vi "Handle Sink Event.vi"(8 "error in (no error)":errorcluster, 10 "Event Data":refnum<class "Event.lvclass">, 11 "Event Source in":refnum<class "Event Source.lvclass">) -> (0 "error out":errorcluster, 3 "Event Source out":refnum<class "Event Source.lvclass">)   [LabVIEW 2016, in "Event Source.lvlib" / "Event Source.lvclass"]
uses:
  Event Source.lvclass
  Event/Event.lvclass
  Event Source Messages/Receive and Broadcast Event Msg/Receive and Broadcast Event Msg.lvclass
  Event Source.lvclass/Event Source.ctl
  Event Source Messages/Abstract Source Event Handler/Abstract Source Event Handler.lvclass
panel:
  in  "Receive and Broadcast Event Msg in":refnum<class "Receive and Broadcast Event Msg.lvclass">
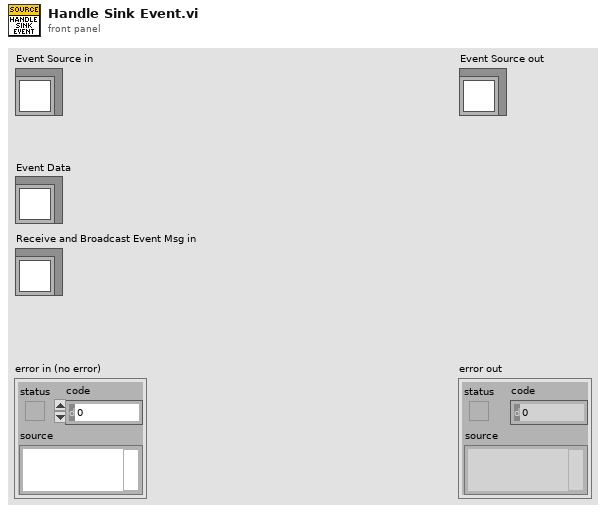
[diagram p1: front panel]
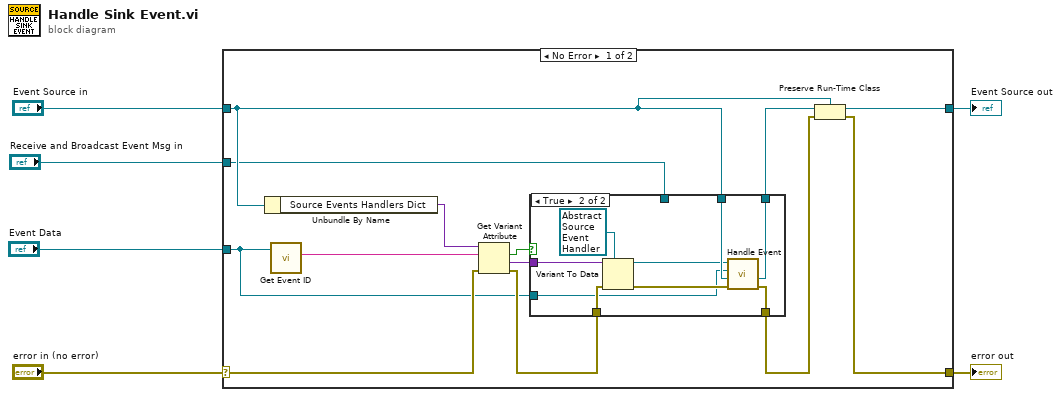
[diagram p0: block diagram]
diagram:
  n1 = case shown="No Error" "error in (no error)" {
    selector: "error in (no error)" -> [w15 w32]
    tunnel: [w9 w32] -> w5
    tunnel: [w12 w31] -> w2
    tunnel: "Event Source in" -> [w11 w31]
    tunnel: "Event Data" -> [w7 _]
    tunnel: "Receive and Broadcast Event Msg in" -> [w8 _]
    frame No Error {
      n2 = Unbundle By Name(w11) -> ("Source Events Handlers Dict"=w19:variant)
      n3 = call-dynamic "Get Event ID.vi"("Event in"=w7) -> ("Event ID"=w18:string)  [unwired: 8 in, 2 out]
      n4 = Get Variant Attribute(Variant=w19, name=w18, error in=w15) -> (found=w17:bool, value=w16:variant, error out=w14:errorcluster)  [unwired: 1 in, 1 out]
      n5 = case shown="True" w17 {
        tunnel: w16 -> [_ w30]
        tunnel: w14 -> [w21 w28]
        tunnel: w11 -> [w20 w24]
        tunnel: [w20 w27] -> w13
        tunnel: [w21 w26] -> w10
        tunnel: w8 -> [_ _]
        tunnel: w7 -> [_ w23]
        frame False {
        }
        frame True {
          n6 = Variant To Data(error in=w28, type=refnum<class "Abstract Source Event Handler.lvclass"> refnum ("Source Event Fire Handler"), Variant=w30) -> (data=w22:refnum<class "Abstract Source Event Handler.lvclass">, error out=w25:errorcluster)
          n7 = call-dynamic "Handle Event.vi"("error in (no error)"=w25, "Event Source in"=w24, "Event Data"=w23, "Abstract Source Event Handler in"=w22) -> ("error out"=w26:errorcluster, "Event Source out"=w27:refnum<class "Event Source.lvclass">)  [unwired: 5 in, 1 out]
        }
      }
      n8 = Preserve Run-Time Class(object in=w13, error in=w10, 2:w11) -> (object out=w12:refnum<class "Event Source.lvclass">, error out=w9:errorcluster)
    }
    frame Error {
    }
  }
  "error out" <- w5
  "Event Source out" <- w2
